vi "View test.vi"() -> ()   [LabVIEW 2015]
panel:
  in  "Array - String":string[](array[string])=["Error", "HTTP", "UDP"]
  out "Array":T1(array[cluster])
  out "Waveform Graph":i32[][](graph)
  in  "File Path Control":path=path "C:/Data/tcp_err.tdms"
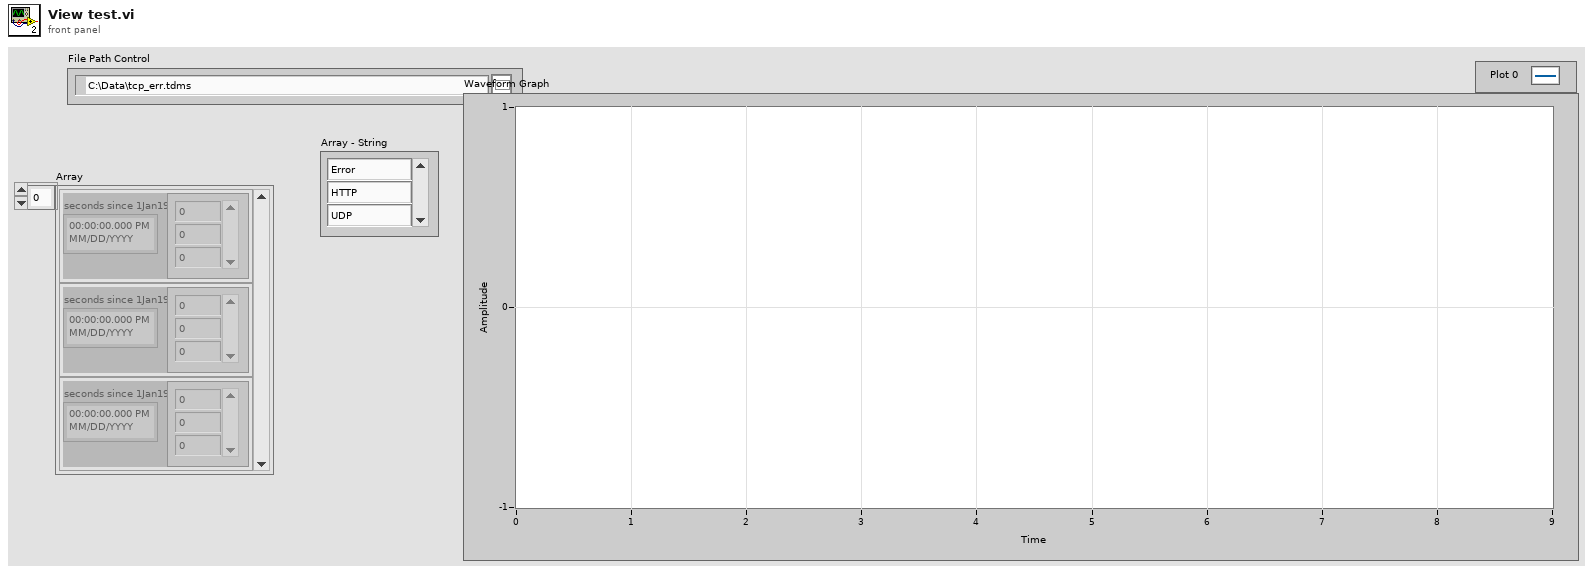
[diagram p1: front panel]
types:
  T1 = cluster{"seconds since 1Jan1904":timestamp, dbl[]}[]
  T2 = cluster{"seconds since 1Jan1904":timestamp, i32[]}
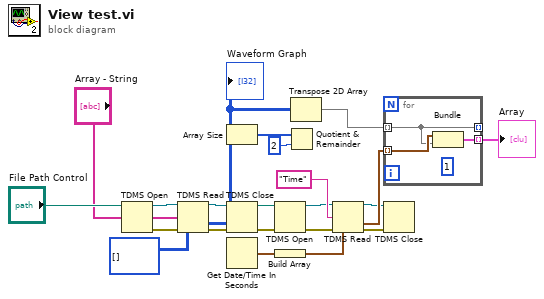
[diagram p0: block diagram]
diagram:
  n1 = TDMS Open(11:"File Path Control") -> (0:w14:errorcluster, 3:w16:refnum<k34>)  [unwired: 6 in]
  n2 = TDMS Read(0:w16, 7:"Array - String", 11:w14, 12:i32[][] []) -> (4:w11:refnum<k34>, 10:w2:i32[][], 15:w13:errorcluster)  [unwired: 4 in, 3 out]
  "Waveform Graph" <- w2
  n3 = Array Size(array=w2) -> (size(s)=w4:i32[])
  n4 = TDMS Close(8:w13, 11:w11) -> (0:w12:errorcluster, 3:w10:path)
  n5 = Get Date/Time In Seconds() -> (seconds since 1Jan1904=w22:timestamp)
  n6 = TDMS Open(8:w12, 11:w10) -> (0:w8:errorcluster, 3:w9:refnum<k34>)  [unwired: 5 in]
  n7 = Build Array(w22) -> (w19:timestamp[])
  n8 = Quotient & Remainder(x=w4, y=2) -> ()  [unwired: 2 out]
  n9 = Transpose 2D Array(2D array=w2) -> (transposed array=w1:i32[][])
  n10 = TDMS Read(0:w9, 7:"Time", 11:w8, 12:w19) -> (4:w15:refnum<k34>, 10:w18:timestamp[], 15:w7:errorcluster)  [unwired: 4 in, 3 out]
  n11 = for {
    tunnel: [w23] -> _ mode=indexing
    tunnel: [w25] -> w5 mode=indexing
    tunnel: w18 -> [w24] mode=indexing
    tunnel: w1 -> [w23] mode=indexing
    (unwired) 1 ("index")
    n12 = Bundle("seconds since 1Jan1904"=w24, w23) -> (w25:T2)  [unwired: 1 in]
  }
  "Array" <- w5
  n13 = TDMS Close(8:w7, 11:w15) -> ()  [unwired: 2 out]
